vi "shootInCloseEnemy.vi"(0 "KickToSkill in":refnum<class "KickToSkill.lvclass">, 1 "robotKickState In":T2=enum."shootFromDirect", 5 "Ball":refnum<class "Ball.lvclass">, 7 "AttackerAngle ToTurnInDegrees":dbl, 9 "EnemyRoboRef":refnum<class "Robot.lvclass">[](array[class]), 11 "error in (no error)":errorcluster, 12 "NewParameters":T1={"PenaltyDistance"=0.0, "DistanceAttackerToBackBall"=0.0, "Division"=enum."Div B", "DistanceToAvoidyEnemyRobot"=0.0, "BallPlacementDistance"=900.0, "DisatanceBehindBallToStealBall"=0.0, "MaxDistanceToPositionKickoff"=2000.0, "BlockEnemyTarget"=FALSE, "MaxStopVAng"=1.0, "DistanceMarkerToEnemy"=0.0, "IgnoreDribblerContact"=FALSE, "DistanceToBeginEnemyPosession"=200.0, "GoToBallWhenEnemyNotMoving"=TRUE, "EnemyDistanceToReduceVelocity"=300.0, "TurnOnEnemyDistanceToReduceVelocity"=TRUE, "EnemyDistanceToShootOutBall"=500.0, "DefenseKickBall"=TRUE, "MoreKickToGoal? (0-0.3)"=0.0, "ChipKickInEnemyField"=TRUE, "ShootOutRobot"=0.0, "FieldLenghtDenominatorInShootOut"=0.0, "GoalieKickForce"=30.0, "AdjustPositionInBallPlacement"=FALSE, "PowerGodPass"=0.0, "VelocityAbortEnemyPos"=0.0, "MaxDistToBeginPass"=500.0, "MinDistToBeginPass"=150.0, "VelocityInDirects"=0.3, "BadDribblerIDs"=[], "NewKickToDistanceAroundBall"=300.0, "PowerAvoidColisionMarker"=0.5, "DistanceToAvoidColisionMarker"=250.0, "AvoidBallKick"=0.0, "DistanceTryKick"=0.0, "SuicideKickDIstance"=0.0, "SuicideKickAtck"=FALSE, "SuicideAngleDistance"=0.0, "SuicideKickDefense"=FALSE, "AvoidAimLessKick"=0.0, "KIckForceWithChipKick"=30.0, "DistanceToAvoidyEnemyShootRobot "=0.0, "NumberOfMarkers"=3.0}, 13 "FieldRef":refnum<class "Field.lvclass">, 14 "Robot in":refnum<class "Robot.lvclass">) -> (4 "KickToSkill out":refnum<class "KickToSkill.lvclass">, 6 "robotKickState out":T2=enum."shootFromDirect", 15 "error out":errorcluster)   [LabVIEW 2020, in "KickToSkill.lvclass"]
uses:
  KickToSkill.lvclass
  Ball_class/Ball.lvclass
  C:/RoboIME/SSL_AI/Object_class/Object.lvclass
  Robot_class/Robot.lvclass
  Robot_class/robotKickToStates.ctl
  Controls/NewParameters.ctl
  Field_class/Field.lvclass
  Object_class/Object.lvclass/Object.ctl
  Robot_class/Robot.lvclass/Robot.ctl
  <vilib>/Analysis/coordinate.llb/Wrap Angle (scalar).vi
  Object_class/Read position(x,y).vi
  Robot_class/Read orientation.vi
  Object_class/Read x.vi
  Robot_class/Read id.vi
  Utilities_class/Utilities.lvclass
  <vilib>/Analysis/NI_AAL_Angle.lvlib
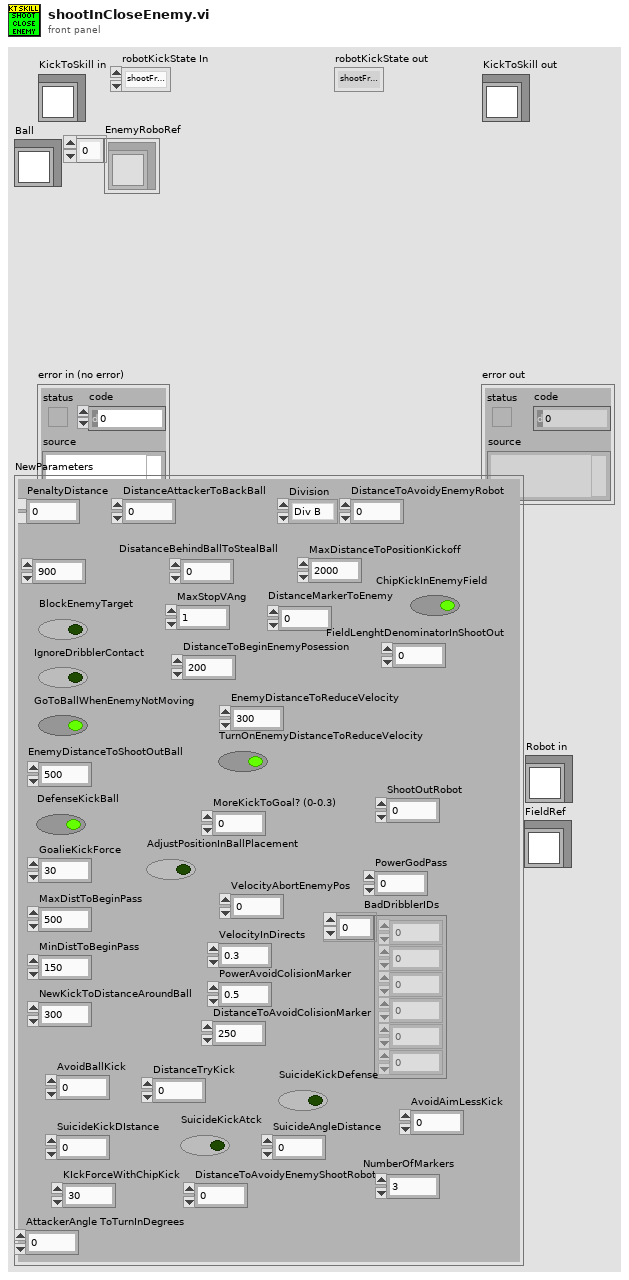
[diagram p1: front panel]
types:
  T1 = typedef "NewParameters.ctl" = cluster{"PenaltyDistance":dbl, "DistanceAttackerToBackBall":dbl, "Division":enum16{"Div B", "Div A"}, "DistanceToAvoidyEnemyRobot":dbl, "BallPlacementDistance":dbl, "DisatanceBehindBallToStealBall":dbl, "MaxDistanceToPositionKickoff":dbl, "BlockEnemyTarget":bool, "MaxStopVAng":dbl, "DistanceMarkerToEnemy":dbl, "IgnoreDribblerContact":bool, "DistanceToBeginEnemyPosession":dbl, "GoToBallWhenEnemyNotMoving":bool, "EnemyDistanceToReduceVelocity":dbl, "TurnOnEnemyDistanceToReduceVelocity":bool, "EnemyDistanceToShootOutBall":dbl, "DefenseKickBall":bool, "MoreKickToGoal? (0-0.3)":dbl, "ChipKickInEnemyField":bool, "ShootOutRobot":dbl, "FieldLenghtDenominatorInShootOut":dbl, "GoalieKickForce":dbl, "AdjustPositionInBallPlacement":bool, "PowerGodPass":dbl, "VelocityAbortEnemyPos":dbl, "MaxDistToBeginPass":dbl, "MinDistToBeginPass":dbl, "VelocityInDirects":dbl, "BadDribblerIDs":i32[], "NewKickToDistanceAroundBall":dbl, "PowerAvoidColisionMarker":dbl, "DistanceToAvoidColisionMarker":dbl, "AvoidBallKick":dbl, "DistanceTryKick":dbl, "SuicideKickDIstance":dbl, "SuicideKickAtck":bool, "SuicideAngleDistance":dbl, "SuicideKickDefense":bool, "AvoidAimLessKick":dbl, "KIckForceWithChipKick":dbl, "DistanceToAvoidyEnemyShootRobot ":dbl, "NumberOfMarkers":dbl}
  T2 = typedef "robotKickToStates.ctl" = enum16{"oldKickTo", "shootFromDirect", "avoidCollideBall", "goToBackBall", "none", "walk", "turn", "shoot"}
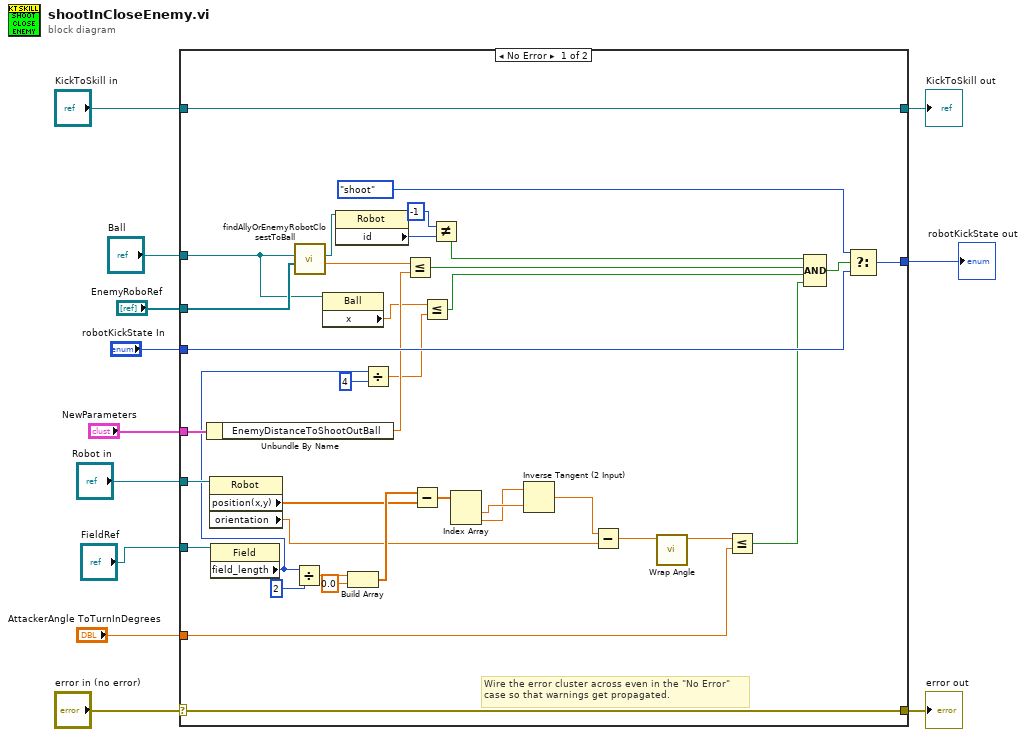
[diagram p0: block diagram]
diagram:
  n1 = case shown="No Error" "error in (no error)" {
    selector: "error in (no error)" -> [w48 w51]
    tunnel: [w48 w51] -> w11
    tunnel: [w49 w50] -> w9
    tunnel: "KickToSkill in" -> [w49 w50]
    tunnel: "Ball" -> [w35 _]
    tunnel: "EnemyRoboRef" -> [w46 _]
    tunnel: "robotKickState In" -> [w39 _]
    tunnel: [w38 _] -> w5
    tunnel: "NewParameters" -> [w37 _]
    tunnel: "Robot in" -> [w33 _]
    tunnel: "FieldRef" -> [w32 _]
    tunnel: "AttackerAngle ToTurnInDegrees" -> [w19 _]
    frame No Error {
      # "Wire the error cluster across even in the \"No Error\"\ncase so that warnings get propagated."
      n2 = Unbundle By Name(w37) -> ("EnemyDistanceToShootOutBall"=w36:dbl)
      n3 = property class="Robot"(reference=w33) -> ("position(x,y)"=w27:dbl[], "orientation"=w22:dbl)  [unwired: 1 in, 2 out]
      n4 = property class="Field"(reference=w32) -> ("field_length"=w16:i32)  [unwired: 1 in, 2 out]
      n5 = Divide(x=w16, y=2) -> (x/y=w30:dbl)
      n6 = call "findAllyOrEnemyRobotClosestToBall.vi"("Ally/Enemy Robots"=w46, "Ball"=w35) -> ("Robot distance to ball"=w47:dbl, "Robot"=w44:refnum<class "Robot.lvclass">)  [unwired: 6 in, 2 out]
      n7 = property class="Ball"(reference=w35) -> ("x"=w17:dbl)  [unwired: 1 in, 2 out]
      n8 = property class="Robot"(reference=w44) -> ("id"=w43:i32)  [unwired: 1 in, 2 out]
      n9 = Build Array(w30, 0.0 ("element")) -> (w28:dbl[])
      n10 = Divide(x=w16, y=4) -> (x/y=w14:dbl)
      n11 = Less Or Equal?(x=w47, y=w36) -> (x <= y?=w45:bool)
      n12 = Subtract(x=w28, y=w27) -> (x-y=w26:dbl[])
      n13 = Less Or Equal?(x=w17, y=w14) -> (x <= y?=w34:bool)
      n14 = Not Equal?(x=-1, y=w43) -> (x != y?=w41:bool)
      n15 = Index Array(array=w26) -> (element #1=w25:dbl, element #2=w24:dbl)  [unwired: 2 in]
      n16 = Inverse Tangent (2 Input)(1:w25, 2:w24) -> (0:w23:dbl)
      n17 = Subtract(x=w23, y=w22) -> (x-y=w21:dbl)
      n18 = call-poly <vilib>:"Wrap Angle.vi"("angle in"=w21) -> ("angle out"=w20:dbl)  [unwired: 9 in, 1 out]
      n19 = Less Or Equal?(x=w20, y=w19) -> (x <= y?=w18:bool)
      n20 = Compound Arithmetic op=AND(w41, w45, w34, w18) -> (w40:bool)
      n21 = Select(t=robotKickToStates."shoot" ("robotKickState"), s=w40, f=w39) -> (s? t:f=w38:T2)
    }
    frame Error {
    }
  }
  "error out" <- w11
  "KickToSkill out" <- w9
  "robotKickState out" <- w5
